vi "IS Open Connection.vi"(8 "error in (no error)":errorcluster, 11 "Access Key":string) -> (0 "error out":errorcluster, 3 "IS Session":T1)   [LabVIEW 2013]
uses:
  <vilib>/httpClient/LabVIEWHTTPClient.lvlib
  <vilib>/httpClient/ClientHandle.ctl
  Custom Data Types/IS Session.ctl
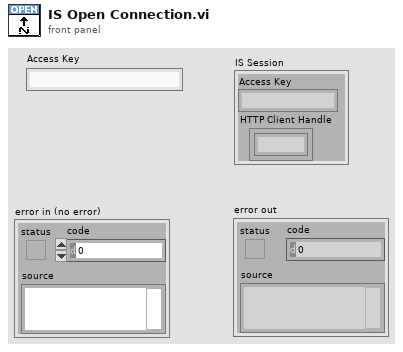
[diagram p1: front panel]
types:
  T1 = typedef "IS Session.ctl" = cluster{"Access Key":string, "HTTP Client Handle":T2}
  T2 = typedef "LabVIEWHTTPClient.lvlib/ClientHandle.ctl" = refnum<k1>
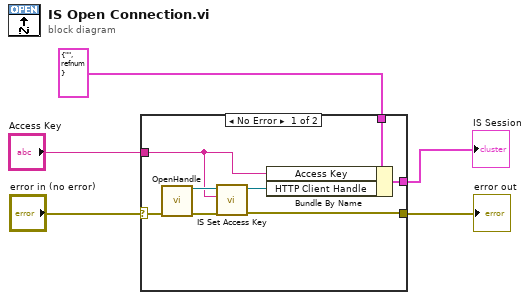
[diagram p0: block diagram]
diagram:
  n1 = case shown="No Error" "error in (no error)" {
    selector: "error in (no error)" -> [w13 w15]
    tunnel: [w6 w15] -> w5
    tunnel: "Access Key" -> [w8 _]
    tunnel: [w12 w14] -> w2
    tunnel: T1 {"Access Key"="", "HTTP Client Handle"=refnum} ("IS Session") -> [w11 w14]
    frame No Error {
      n2 = call <vilib>:"OpenHandle.vi"("error in (no error)"=w13) -> ("client handle out"=w10:T2, "error out"=w9:errorcluster)  [unwired: 13 in]
      n3 = call "IS Set Access Key.vi"("HTTP Client Handle in"=w10, "Access Key"=w8, "error in (no error)"=w9) -> ("HTTP Client Handle out"=w7:T2, "error out"=w6:errorcluster)  [unwired: 6 in]
      n4 = Bundle By Name(cluster=w11, "Access Key"=w8, "HTTP Client Handle"=w7) -> (w12:T1)
    }
    frame Error {
    }
  }
  "error out" <- w5
  "IS Session" <- w2
